vi "Lesson 1- booleans.vi"() -> ()   [LabVIEW 2024]
panel:
  out "iteration":i32
  in  "wait (ms)":u32=10
  out "a implies b 2":bool[](array[boolean])=[TRUE, FALSE, TRUE, TRUE]
  out "8bit integer (hex)":i8=39 format="%0x"
  out "unsigned 8bit integer (hex)":u8=39 format="%0x"
  out "8bit integer":i8=39
  out "unsigned 8bit integer":u8=39
  in  "offset":i32=-128
  out "signed":bool[](array[boolean])=[TRUE, TRUE, TRUE, FALSE, FALSE, TRUE, FALSE, FALSE]
  out "unsigned":bool[](array[boolean])=[TRUE, TRUE, TRUE, FALSE, FALSE, TRUE, FALSE, FALSE]
  in  "Loop For N":i32=256
  out "8-bit count":bool[][](array[boolean])=[[FALSE, FALSE, FALSE, FALSE, FALSE, FALSE, FALSE, FALSE], [TRUE, FALSE, FALSE, FALSE, FALSE, FALSE, FALSE, FALSE], [FALSE, TRUE, FALSE, FALSE, FALSE, FALSE, FALSE, FALSE], [TRUE, TRUE, FALSE, FALSE, FALSE, FALSE, FALSE, FALSE]]
  out "32-bit count":bool[][](array[boolean])=[[FALSE, FALSE, FALSE, FALSE, FALSE, FALSE, FALSE, FALSE, FALSE, FALSE, FALSE, FALSE, FALSE, FALSE, FALSE, FALSE, FALSE, FALSE, FALSE, FALSE, FALSE, FALSE, FALSE, FALSE, FALSE, FALSE, FALSE, FALSE, FALSE, FALSE, FALSE, FALSE], [TRUE, FALSE, FALSE, FALSE, FALSE, FALSE, FALSE, FALSE, FALSE, FALSE, FALSE, FALSE, FALSE, FALSE, FALSE, FALSE, FALSE, FALSE, FALSE, FALSE, FALSE, FALSE, FALSE, FALSE, FALSE, FALSE, FALSE, FALSE, FALSE, FALSE, FALSE, FALSE], [FALSE, TRUE, FALSE, FALSE, FALSE, FALSE, FALSE, FALSE, FALSE, FALSE, FALSE, FALSE, FALSE, FALSE, FALSE, FALSE, FALSE, FALSE, FALSE, FALSE, FALSE, FALSE, FALSE, FALSE, FALSE, FALSE, FALSE, FALSE, FALSE, FALSE, FALSE, FALSE], [TRUE, TRUE, FALSE, FALSE, FALSE, FALSE, FALSE, FALSE, FALSE, FALSE, FALSE, FALSE, FALSE, FALSE, FALSE, FALSE, FALSE, FALSE, FALSE, FALSE, FALSE, FALSE, FALSE, FALSE, FALSE, FALSE, FALSE, FALSE, FALSE, FALSE, FALSE, FALSE]]
  out "a implies b":bool[](array[boolean])=[TRUE, FALSE, TRUE, TRUE]
  out "a xnor b":bool[](array[boolean])=[TRUE, FALSE, FALSE, TRUE]
  out "a nor b":bool[](array[boolean])=[TRUE, FALSE, FALSE, FALSE]
  out "a nand b":bool[](array[boolean])=[TRUE, TRUE, TRUE, FALSE]
  out "a xor b":bool[](array[boolean])=[FALSE, TRUE, TRUE, FALSE]
  out "a or b":bool[](array[boolean])=[FALSE, TRUE, TRUE, TRUE]
  out "a and b":bool[](array[boolean])=[FALSE, FALSE, FALSE, TRUE]
  in  "b":bool[](array[boolean])=[FALSE, FALSE, TRUE, TRUE]
  in  "a":bool[](array[boolean])=[FALSE, TRUE, FALSE, TRUE]
  out ".not. x?":bool
  out "x out":bool=TRUE
  in  "x":bool=TRUE
  # "Also covered:\n* Arrays\n* For Loop\n* Signed and Unsigned Intergers\n* Basic timing delay\n* Number to Array"
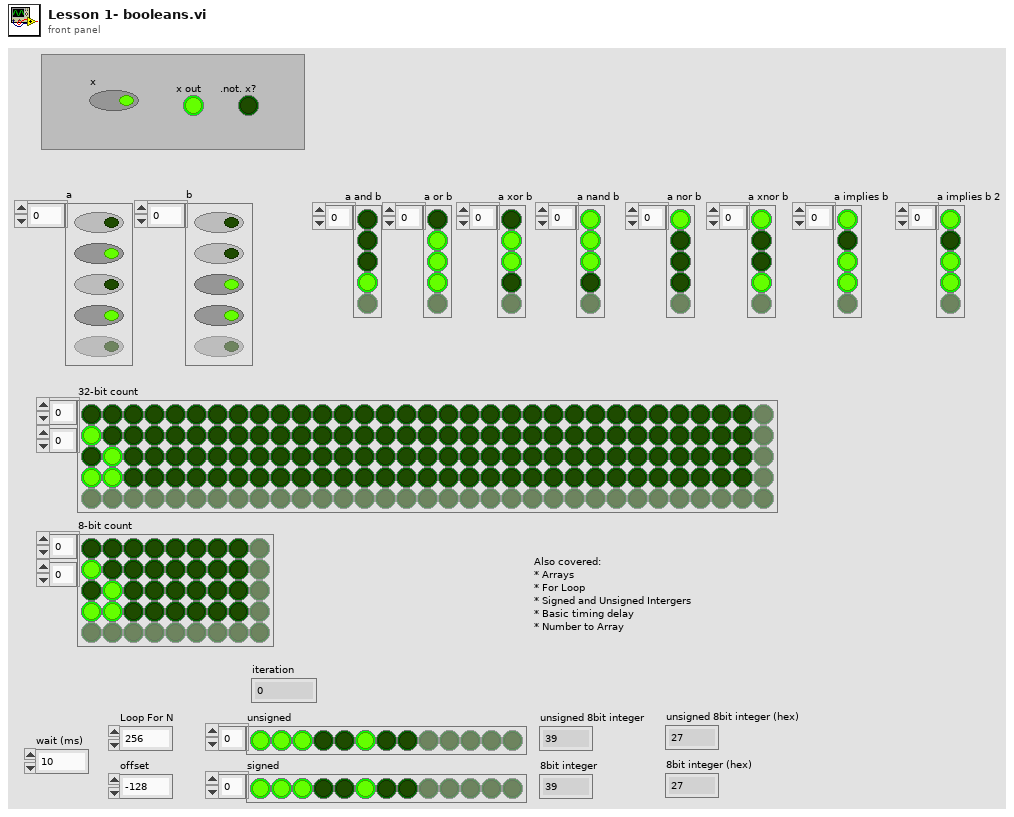
[diagram p1: front panel]
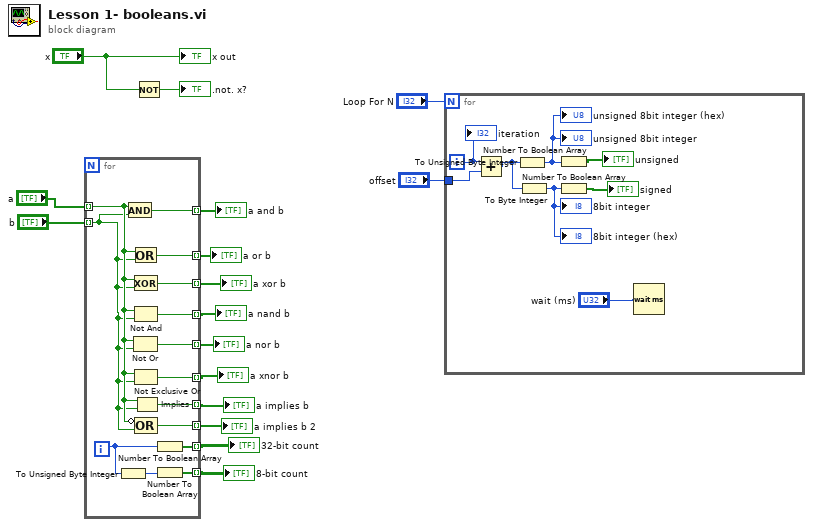
[diagram p0: block diagram]
diagram:
  n1 = for {
    tunnel: "a" -> [w19] mode=indexing
    tunnel: "b" -> [w18] mode=indexing
    tunnel: [w30] -> w13 mode=indexing
    tunnel: [w29] -> w12 mode=indexing
    tunnel: [w28] -> w11 mode=indexing
    tunnel: [w27] -> w10 mode=indexing
    tunnel: [w26] -> w9 mode=indexing
    tunnel: [w25] -> w8 mode=indexing
    tunnel: [w24] -> w7 mode=indexing
    tunnel: [w23] -> w5 mode=indexing
    tunnel: [w20] -> w4 mode=indexing
    tunnel: [w17] -> w1 mode=indexing
    i -> [w22]
    n2 = To Unsigned Byte Integer(number=w22) -> (unsigned 8bit integer=w21:u8)
    n3 = And(x=w19, y=w18) -> (x .and. y?=w30:bool)
    n4 = Not Or(1:w18, 2:w19) -> (0:w26:bool)
    n5 = Or(x=w19, y=w18) -> (x .or. y?=w29:bool)
    n6 = Exclusive Or(1:w18, 2:w19) -> (0:w28:bool)
    n7 = Not And(1:w18, 2:w19) -> (0:w27:bool)
    n8 = Not Exclusive Or(1:w18, 2:w19) -> (0:w25:bool)
    n9 = Implies(1:w18, 2:w19) -> (0:w24:bool)
    n10 = Compound Arithmetic op=OR(invert w19, w18) -> (w17:bool)
    n11 = Number To Boolean Array(number=w22) -> (Boolean array=w23:bool[])
    n12 = Number To Boolean Array(number=w21) -> (Boolean array=w20:bool[])
  }
  "a and b" <- w13
  "a or b" <- w12
  "a xor b" <- w11
  "a nand b" <- w10
  "a nor b" <- w9
  "a xnor b" <- w8
  "a implies b" <- w7
  "32-bit count" <- w5
  "8-bit count" <- w4
  "a implies b 2" <- w1
  n13 = Not(x="x") -> (.not. x?=→".not. x?":bool)
  n14 = for {
    N: "Loop For N" -> [_]
    tunnel: "offset" -> [w35]
    i -> [w31]
    n15 = Add(x=w31, y=w35) -> (x+y=w36:i32)
    n16 = To Unsigned Byte Integer(number=w36) -> (unsigned 8bit integer=w34:u8)
    "unsigned 8bit integer" <- w34
    "unsigned 8bit integer (hex)" <- w34
    n17 = To Byte Integer(number=w36) -> (8bit integer=w33:i8)
    "8bit integer" <- w33
    "8bit integer (hex)" <- w33
    n18 = Number To Boolean Array(number=w34) -> (Boolean array=→"unsigned":bool[])
    n19 = Number To Boolean Array(number=w33) -> (Boolean array=→"signed":bool[])
    n20 = Wait (ms)(milliseconds to wait="wait (ms)") -> ()  [unwired: 1 out]
    "iteration" <- w31
  }
  "x out" <- "x"
